vi "XOR Encryption - (2) Sender and Receiver Have Separate Keys.vi"() -> ()   [LabVIEW 2013]
panel:
  out "Data Out":string
  in  "Data In":string
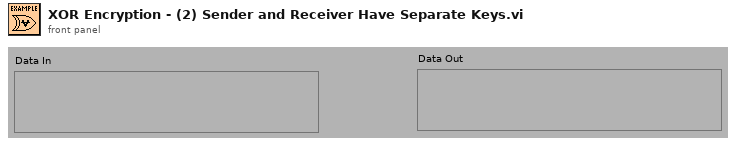
[diagram p1: front panel]
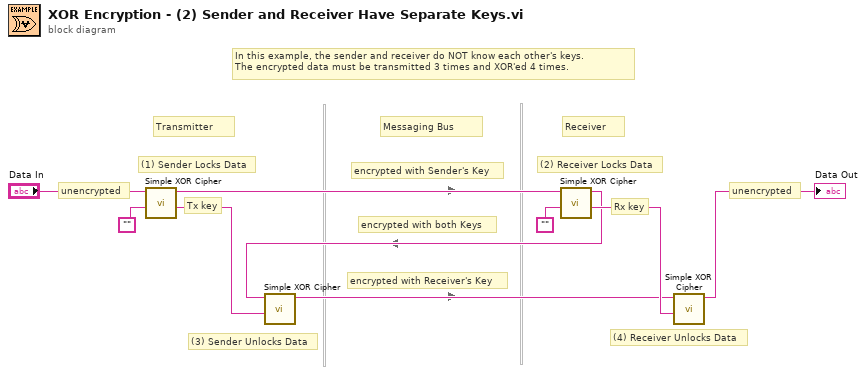
[diagram p0: block diagram]
diagram:
  # "Messaging Bus"
  # "Receiver"
  # "Transmitter"
  # "unencrypted"
  # "unencrypted"
  # "Rx key"
  # "Tx key"
  # "In this example, the sender and receiver do NOT know each other's keys.\nThe encrypted data must be transmitted 3 times and XOR'ed 4 times."
  # "encrypted with Receiver's Key"
  # "encrypted with Sender's Key"
  # "encrypted with both Keys"
  # "(4) Receiver Unlocks Data"
  # "(3) Sender Unlocks Data"
  # "(2) Receiver Locks Data"
  # "(1) Sender Locks Data"
  n1 = call "Simple XOR Cipher.vi"("key (\"\": random)"="", "data in"="Data In") -> ("key out"=w6:string, "data out"=w3:string)  [unwired: 8 in]
  n2 = call "Simple XOR Cipher.vi"("key (\"\": random)"="", "data in"=w3) -> ("key out"=w7:string, "data out"=w1:string)  [unwired: 8 in]
  n3 = call "Simple XOR Cipher.vi"("key (\"\": random)"=w6, "data in"=w1) -> ("data out"=w2:string)  [unwired: 8 in, 1 out]
  n4 = call "Simple XOR Cipher.vi"("key (\"\": random)"=w7, "data in"=w2) -> ("data out"=→"Data Out":string)  [unwired: 8 in, 1 out]
